vi "Init.vi"(10 "jettl":refnum<class "jettl.lvclass">) -> (3 "Last Ack Creator Msg Strategy out":refnum<class "Last Ack Creator Msg Strategy.lvclass">)   [LabVIEW 2021, in "jettl.lvlib" / "Last Ack Creator Msg Strategy.lvlib" / "Last Ack Creator Msg Strategy.lvclass"]
uses:
  Last Ack Creator Msg Strategy.lvclass
  jettl/jettl.lvclass
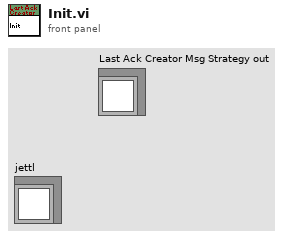
[diagram p1: front panel]
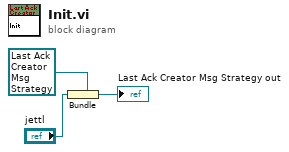
[diagram p0: block diagram]
diagram:
  n1 = Bundle "Bundle"(cluster=refnum<class "Last Ack Creator Msg Strategy.lvclass"> refnum ("Last Ack Creator Queue Msg Strategy out"), "jettl") -> (→"Last Ack Creator Msg Strategy out":refnum<class "Last Ack Creator Msg Strategy.lvclass">)
